vi "sub_get-motion-model.vi"(3 "motion":cluster{"x":dbl, "y":dbl}[](array[cluster])=[{"x"=1.0, "y"=0.0}, {"x"=0.0, "y"=1.0}, {"x"=-1.0, "y"=0.0}, {"x"=0.0, "y"=-1.0}, {"x"=-1.0, "y"=-1.0}, {"x"=-1.0, "y"=1.0}, {"x"=1.0, "y"=-1.0}, {"x"=1.0, "y"=1.0}]) -> ()   [LabVIEW 2019]
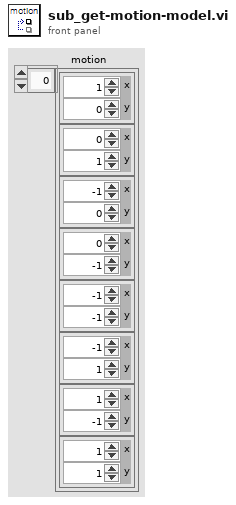
[diagram p1: front panel]
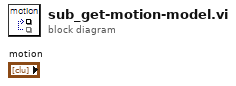
[diagram p0: block diagram]
diagram:
